vi "nanomsg_recv_multi.vi"(3 "error in":errorcluster, 4 "no block? (F)":bool, 5 "socket in":refnum<class "nanomsg_socket.lvclass">) -> (0 "error out":errorcluster, 1 "parts":string[](array[string]), 2 "socket out":refnum<class "nanomsg_socket.lvclass">)   [LabVIEW 2014]
doc: "Receive a multi-component message from the socket. The incoming messages are returned as an array of strings, with one string for each message part.\n\nIf <b>no block?</b> is True, the function call will return immediately. \n\nOtherwise this call will block until <b>all</b> parts of the message are received, an error is raised, or the socket is closed.\n\nNote there is no penalty using this function to receive single-part messages."
uses:
  nanomsg.lvlib
  nanomsg_socket.lvclass
panel:
  # "NN"
  # "labview"
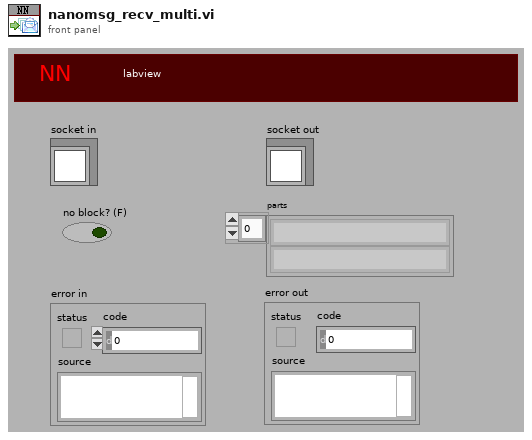
[diagram p1: front panel]
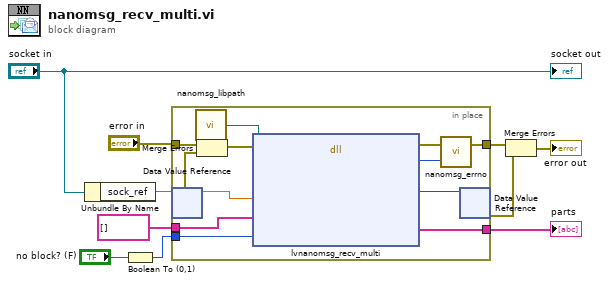
[diagram p0: block diagram]
diagram:
  n1 = Unbundle By Name("socket in") -> ("sock_ref"=w6)
  n2 = Boolean To (0,1)(Boolean="no block? (F)") -> (0, 1=w1:i16)
  n3 = in-place {
    in-place-border: "error in" -> [w20]
    in-place-border: [w19] -> w9
    in-place-border: string[] [] ("parts") -> [w18]
    in-place-border: [w15] -> w5
    in-place-border: w1 -> [w11]
    n4 = in-place-dvr #1(w6) -> (w17:dbl, w12:errorcluster)
    n5 = call "nanomsg_libpath.vi"() -> ("path"=w14:path)
    n6 = Merge Errors(w20, w12) -> (w13:errorcluster)
    n7 = dll-call lib="?" fn="lvnanomsg_recv_multi" ("zmq_labview.dll:lvzmq_socket")(path in=w14, error in=w13, "sock_obj"=w17, "data"=w18, "flags"=w11) -> (error out=w22:errorcluster, "return type"=w21:i32, "sock_obj"=w16:u64, "data"=w15:string[])  [unwired: 4 in, 1 out]
    n8 = call "nanomsg_errno.vi"("retval"=w21, "error in"=w22) -> ("error out"=w19:errorcluster)  [unwired: 1 out]
    n9 = in-place-dvr #1(w16) -> (w3:errorcluster)  [unwired: 1 out]
  }
  "parts" <- w5
  n10 = Merge Errors(w9, w3) -> (→"error out":errorcluster)
  "socket out" <- "socket in"
